vi "isCancelled.vi"(8 "error in (no error)":errorcluster, 11 "GRPCMessage in":refnum<class "GRPCMessage.lvclass">) -> (0 "error out":errorcluster, 2 "isCancelled?":bool, 3 "GRPCMessage out":refnum<class "GRPCMessage.lvclass">)   [LabVIEW 2019, in "MicronGRPCServer.lvlib" / "GRPCMessage.lvclass"]
uses:
  GRPCMessage.lvclass
  GRPCMessage.lvclass/GRPCMessage.ctl
  <vilib>/gRPC/LabVIEW gRPC Library/grpc-lvsupport-release.lvlib
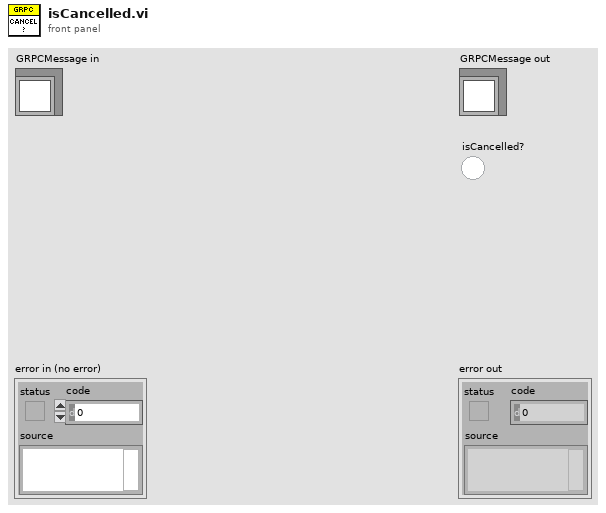
[diagram p1: front panel]
types:
  T1 = typedef "grpc-lvsupport-release.lvlib/grpcId.ctl" = u64
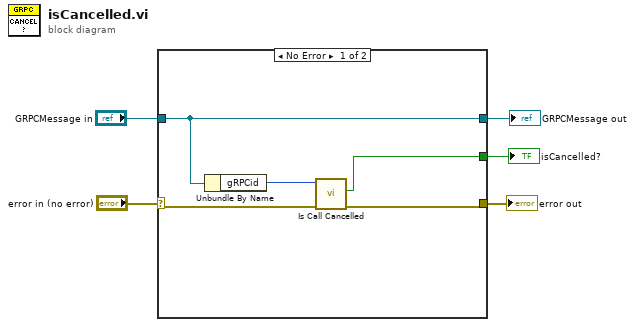
[diagram p0: block diagram]
diagram:
  n1 = case shown="No Error" "error in (no error)" {
    selector: "error in (no error)" -> [w10 w12]
    tunnel: [w9 w12] -> w4
    tunnel: "GRPCMessage in" -> [w8 w11]
    tunnel: [w8 w11] -> w2
    tunnel: [w6 _] -> w1
    frame No Error {
      n2 = Unbundle By Name(w8) -> ("gRPCid"=w7:T1)
      n3 = call <vilib>:"Is Call Cancelled.vi"("error in"=w10, "gRPCid in"=w7) -> ("error out"=w9:errorcluster, "Is Cancelled"=w6:bool)  [unwired: 7 in, 1 out]
    }
    frame Error {
    }
  }
  "error out" <- w4
  "GRPCMessage out" <- w2
  "isCancelled?" <- w1
